vi "array to data claster.vi"(11 "Array":u64[](array[numeric])) -> (3 "Cluster":T1={"PW"=0, "frequency shift"=0.0, "amp"=0.9999923706054688, "mode type"=enum."CW", "mode depth"=0, "mode filter"=0})   [LabVIEW 2021]
doc: "convert compresed data to PDW for the DDS"
uses:
  pdw.ctl
  mode_type.ctl
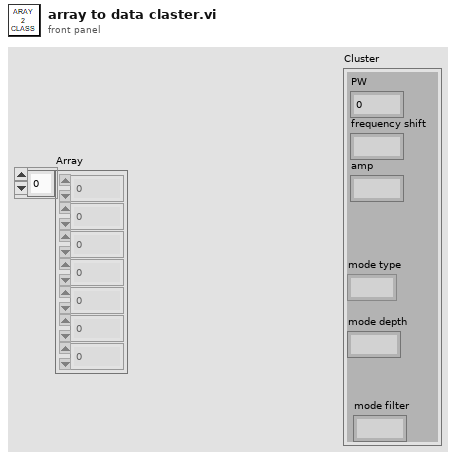
[diagram p1: front panel]
types:
  T1 = typedef "pdw.ctl" = cluster{"PW":u32, "frequency shift":fxp<+/-,48,0>, "amp":fxp<+/-,18,1>, "mode type":T2, "mode depth":u32, "mode filter":u8}
  T2 = typedef "mode_type.ctl" = enum8{"CW", "NC - CW", "NC - cw", "LFM", "BPSK", "QPSK"}
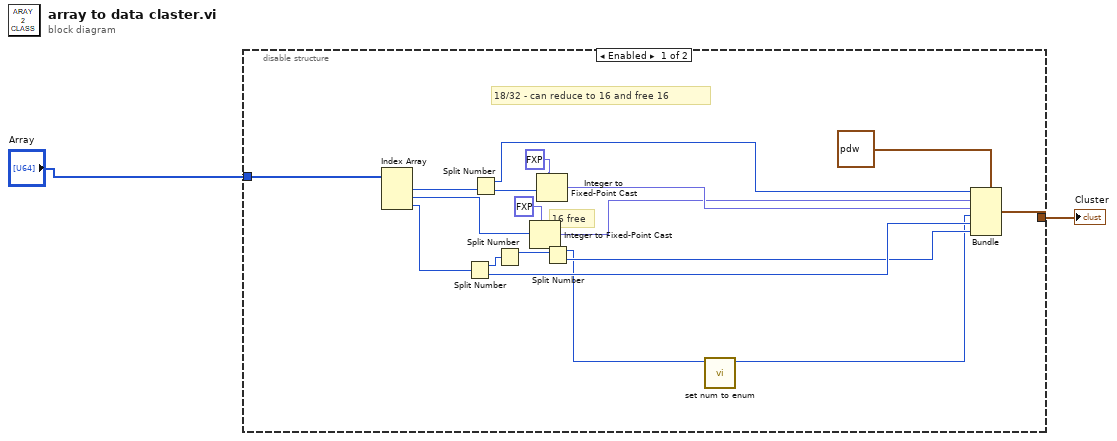
[diagram p0: block diagram]
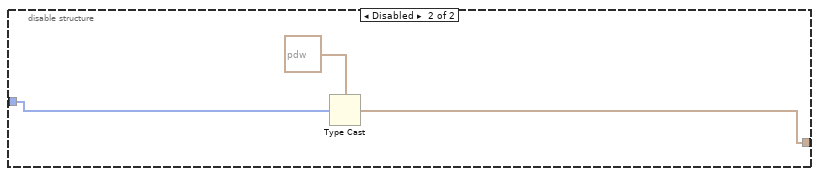
[diagram p2: hidden frame]
diagram:
  n1 = disable-structure shown="Enabled" {
    disable-tunnel: "Array" -> [w15 w22]
    disable-tunnel: [w13 w21] -> w1
    frame Enabled {
      # "16 free"
      # "18/32 - can reduce to 16 and free 16"
      n2 = Index Array(array=w15) -> (element #1=w16:u64, element #2=w18:u64, element #3=w9:u64)  [unwired: 3 in]
      n3 = Split Number(x=w9) -> (hi(x)=w7:u32, lo(x)=w8:u32)
      n4 = Split Number(x=w16) -> (hi(x)=w12:u32, lo(x)=w20:u32)
      n5 = Split Number(x=w7) -> (hi(x)=w6:u16)  [unwired: 1 out]
      n6 = Integer to Fixed-Point Cast(fixed-point type=fxp<+/-,48,0> 0.0 ("frequency shift"), integer=w18) -> (fixed-point=w10:fxp<+/-,48,0>)
      n7 = Integer to Fixed-Point Cast(fixed-point type=fxp<+/-,18,1> 0.0 ("I"), integer=w20) -> (fixed-point=w11:fxp<+/-,18,1>)
      n8 = Split Number(x=w6) -> (hi(x)=w4:u8, lo(x)=w5:u8)
      n9 = call "set num to enum.vi"("Numeric in"=w4) -> ("Numeric out"=w3:T2)  [unwired: 10 in]
      n10 = Bundle(cluster=T1 {"PW"=0, "frequency shift"=0.0, "amp"=0.9999923706054688, "mode type"=enum."CW", "mode depth"=0, "mode filter"=0} ("Cluster"), "PW"=w12, "frequency shift"=w10, "amp"=w11, "mode type"=w3, "mode depth"=w8, "mode filter"=w5) -> (w13:T1)
    }
    frame Disabled {
      n11 = Type Cast(type=T1 {"PW"=0, "frequency shift"=0.0, "amp"=0.9999923706054688, "mode type"=enum."CW", "mode depth"=0, "mode filter"=0} ("Cluster"), x=w22) -> (*(type *) &x=w21:T1)
    }
  }
  "Cluster" <- w1
